vi "Autonomous Independent.vi"() -> ()   [LabVIEW 2016]
doc: "This VI is called when autonomous begins, and will automatically be terminated when autonomous ends. You can carry out timed or sensor driven robot movement independently without needing to return to the caller."
uses:
  <vilib>/Rock Robotics/WPI/Solenoid/WPI_SolenoidValue.ctl
  <vilib>/Rock Robotics/WPI/Utilities/WPI_GetSetVariantRefNum.vi
  <vilib>/Rock Robotics/Network Tables/NT Write Numeric Array.vi
  <vilib>/Rock Robotics/Network Tables/NT Read String.vi
  <vilib>/Rock Robotics/WPI/Solenoid/WPI_SolenoidSetEnum.vi
  <vilib>/addons/control/pid/pid.llb/PID (DBL).vi
  <vilib>/Rock Robotics/WPI/RobotDrive/WPI_RobotDriveMecanumDrive_Cartesian.vi
  <vilib>/Rock Robotics/Network Tables/NT Read Number.vi
  <vilib>/addons/control/pid/NI_PID_pid.lvlib
panel:
  out "Elapsed Time (s) 3":dbl caption="Elapsed Time (s)"
  out "Time has Elapsed 3":bool caption="Time has Elapsed"
  out "s? t:f 3":dbl=0.9
  out "x .or. y? 3":bool=TRUE
  in  "speed 3":dbl(slide)=0.10126903553299492 scale=-0.15..0.15
  in  "setpoint 3":dbl(slide) scale=-50.0..50.0
  in  "PID gains 3":T1={"proportional gain (Kc)"=1.0, "integral time (Ti, min)"=0.01, "derivative time (Td, min)"=0.0} {"derivative time (Td, min)" scale=0.0..0.05; "integral time (Ti, min)" scale=0.0..0.00243; "proportional gain (Kc)" scale=0.0..0.284195}
  out "proportional gain (Kc) 3":dbl=1.0
  out "integral time (Ti, min) 3":dbl=0.01
  out "derivative time (Td, min) 3":dbl
  out "substitute 3":bool
  out "STOP? 3":bool
  out "limit of sensor dist 3":dbl
  out "Current Movement, for debugging":T2 {"Z Joystick Value" scale=-1.0..1.0; "Y Joystick Value" scale=1.0..-1.0; "X Joystick Value" scale=-1.0..1.0}
  in  "Array of robot movements":T3(array[cluster])=[{"X Joystick Value"=-0.010101010101010017, "Y Joystick Value"=0.0, "Z Joystick Value"=0.4574773480918073, "Delay (sec)"=0.0, "Movement Name"=""}, {"X Joystick Value"=0.050505050505050594, "Y Joystick Value"=0.0, "Z Joystick Value"=-0.25616029503917137, "Delay (sec)"=0.0, "Movement Name"=""}] {"Z Joystick Value" scale=-1.0..1.0; "Y Joystick Value" scale=1.0..-1.0; "X Joystick Value" scale=-1.0..1.0}
  out "Elapsed Time (s) 2":dbl caption="Elapsed Time (s)"
  out "Time has Elapsed 2":bool caption="Time has Elapsed"
  out "s? t:f 2":dbl=0.9
  out "x .or. y? 2":bool=TRUE
  in  "speed 2":dbl(slide)=0.10126903553299492 scale=-0.15..0.15
  in  "setpoint 2":dbl(slide) scale=-50.0..50.0
  in  "PID gains 2":T1={"proportional gain (Kc)"=1.0, "integral time (Ti, min)"=0.01, "derivative time (Td, min)"=0.0} {"derivative time (Td, min)" scale=0.0..0.05; "integral time (Ti, min)" scale=0.0..0.00243; "proportional gain (Kc)" scale=0.0..0.284195}
  out "proportional gain (Kc) 2":dbl=1.0
  out "integral time (Ti, min) 2":dbl=0.01
  out "derivative time (Td, min) 2":dbl
  out "substitute 2":bool
  out "STOP? 2":bool
  out "limit of sensor dist 2":dbl
  out "Elapsed Time (s)":dbl
  out "Time has Elapsed":bool
  out "Left":dbl(graph)=57.45456942754214
  out "Right":dbl(graph)=69.75220843172497
  out "s? t:f":dbl=0.9
  out "x .or. y?":bool=TRUE
  in  "speed":dbl(slide)=0.10126903553299492 scale=-0.15..0.15
  out "Yaw":dbl(graph)
  out "Data":T4(graph)={"setpoint"=0.0, "Yaw"=2.26, "dt out (s)"=0.0010000000474974513}
  in  "setpoint":dbl(slide) scale=-50.0..50.0
  in  "PID gains":T1={"proportional gain (Kc)"=1.0, "integral time (Ti, min)"=0.01, "derivative time (Td, min)"=0.0} {"derivative time (Td, min)" scale=0.0..0.05; "integral time (Ti, min)" scale=0.0..0.00243; "proportional gain (Kc)" scale=0.0..0.284195}
  out "proportional gain (Kc)":dbl=1.0
  out "integral time (Ti, min)":dbl=0.01
  out "derivative time (Td, min)":dbl
  out "substitute":bool
  out "Right Average":cluster{dbl}(graph)
  out "Left Average":cluster{dbl}(graph)
  out "STOP?":bool
  out "limit of sensor dist":dbl
  out "Yaw 2":dbl
  out "Yaw 3":dbl
  # "Be sure to right-click and choose Data Operations>>Make Current Value default if you want to save the array values with the VI"
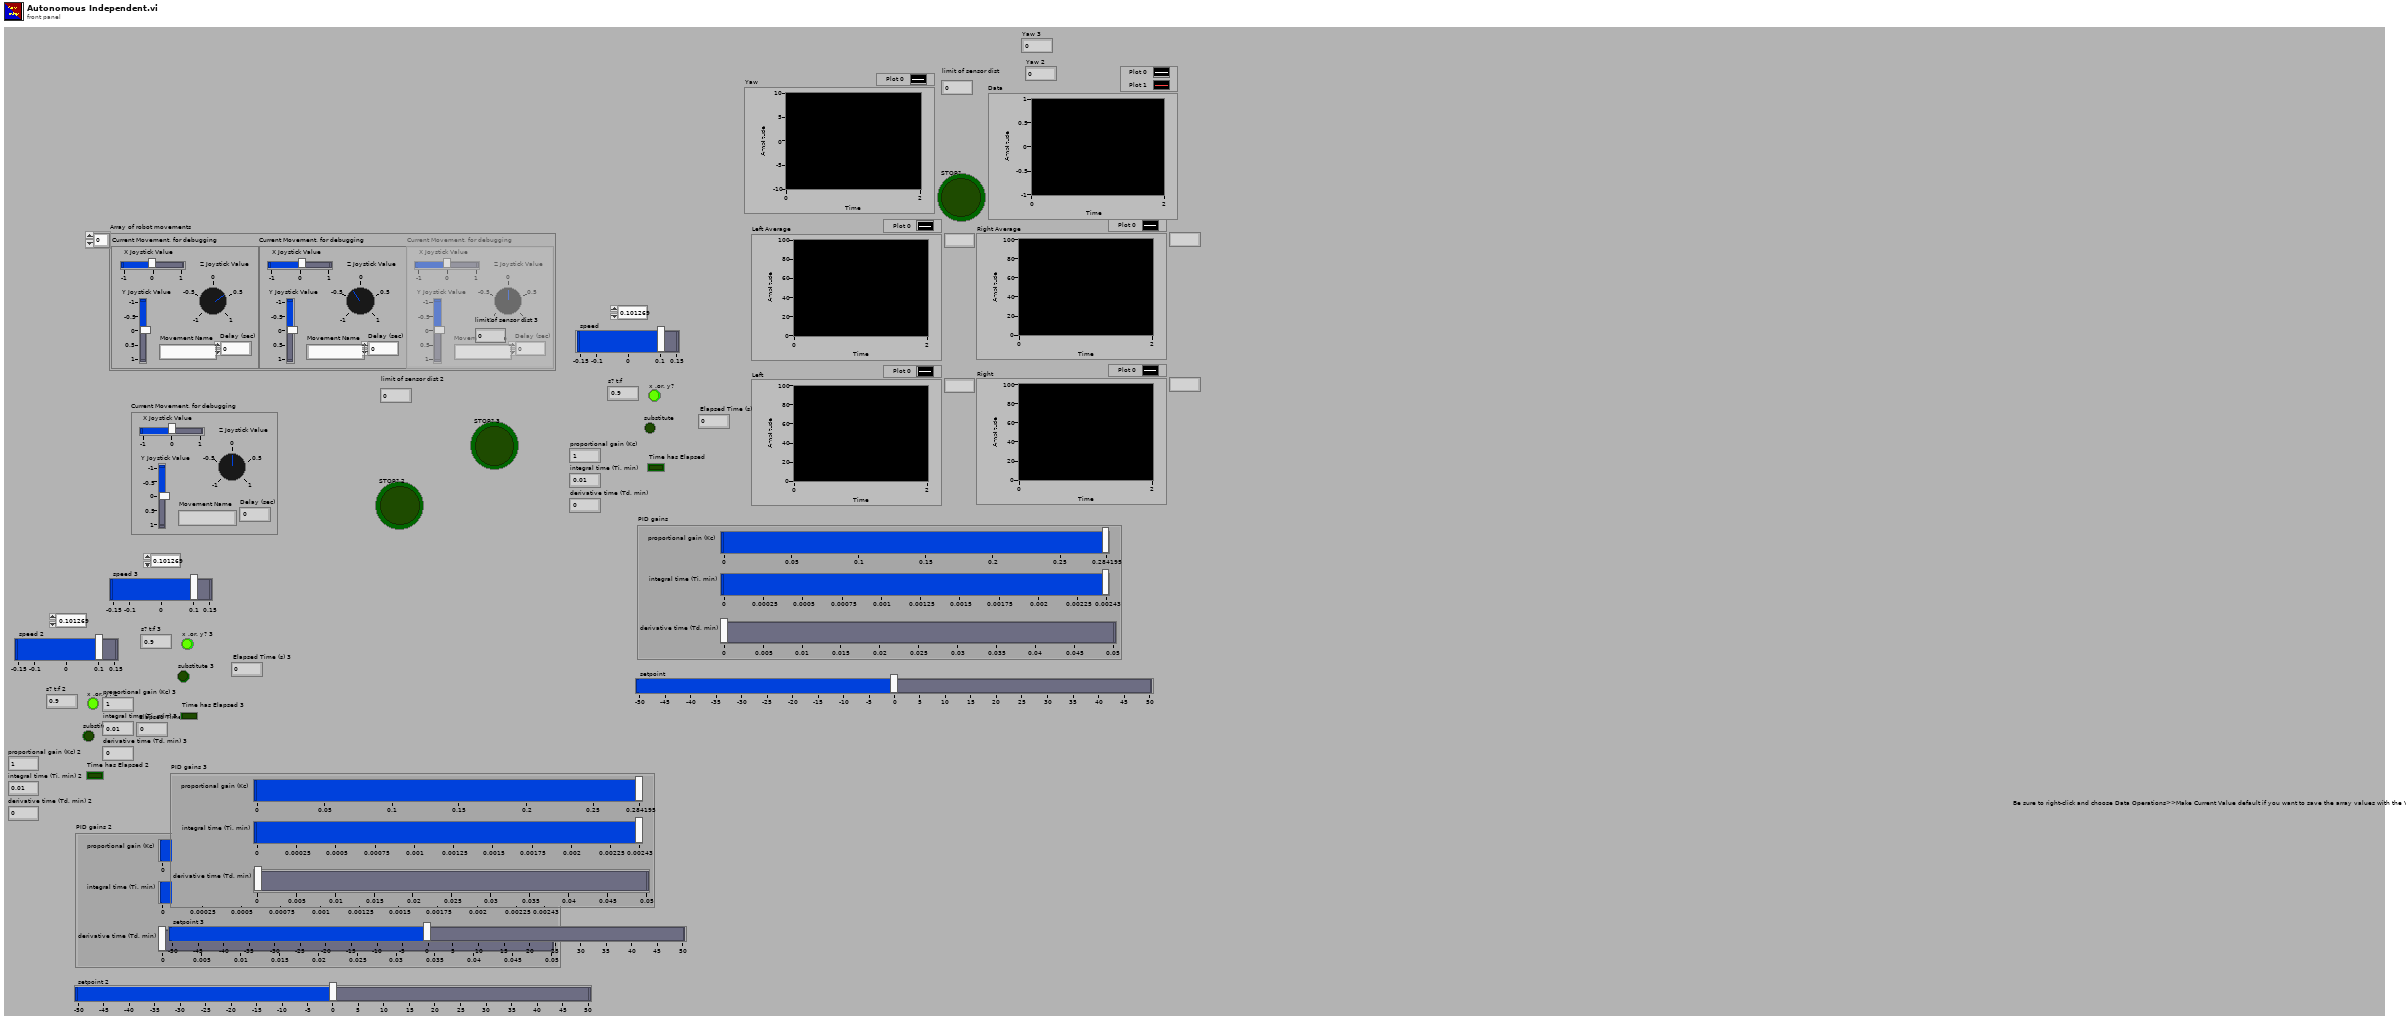
[diagram p1: front panel]
types:
  T1 = cluster{"proportional gain (Kc)":dbl, "integral time (Ti, min)":dbl, "derivative time (Td, min)":dbl}
  T2 = cluster{"X Joystick Value":dbl, "Y Joystick Value":dbl, "Z Joystick Value":dbl, "Delay (sec)":dbl, "Movement Name":string}
  T3 = cluster{"X Joystick Value":dbl, "Y Joystick Value":dbl, "Z Joystick Value":dbl, "Delay (sec)":dbl, "Movement Name":string}[]
  T4 = cluster{"setpoint":dbl, "Yaw":dbl, "dt out (s)":dbl}
  T5 = typedef "WPI_JoystickDevRef.ctl" = cluster{"Device":T6}
  T6 = typedef "WPI_JoystickDeviceEnum.ctl" = enum16{"USB 0", "USB 1", "USB 2", "USB 3", "USB 4", "USB 5"}
  T7 = typedef "WPI_SolenoidValue.ctl" = enum16{"Off", "On", "Forward", "Reverse"}
  T8 = typedef "WPI_SolenoidDevRef.ctl" = cluster{"DevStatus":errorcluster, "Pneumatics Control Module":u8, "Forward Solenoid Channel":T9, "Reverse Solenoid Channel":T9}
  T9 = typedef "WPI_SolenoidChannel.ctl" = enum8{"Solenoid 0", "Solenoid 1", "Solenoid 2", "Solenoid 3", "Solenoid 4", "Solenoid 5", "Solenoid 6", "Solenoid 7", "Invalid"}
  T10 = typedef "WPI_AnalogChannelDevRef.ctl" = cluster{"DevStatus":errorcluster, "Analog Channel":T11}
  T11 = typedef "FPGA_AIChannel.ctl" = enum8{"AI 0", "AI 1", "AI 2", "AI 3", "AI MXP 0", "AI MXP 1", "AI MXP 2", "AI MXP 3", "Invalid"}
  T12 = typedef "WPI_RobotDriveDevRef.ctl" = cluster{"DevStatus":errorcluster, "Motors[]":T13[], "Square Inputs":bool, "Max Output":dbl}
  T13 = typedef "WPI_MotorControlDeviceRef.ctl" = cluster{"DeviceStatus":errorcluster, "Type":T14, "PWM":cluster{"PWM Channel":T15, "DeadBand":T16}, "CAN":cluster{"Device Number":u8, "SetOutput VI Ref":variant, "GetOutput VI Ref":variant, "Enable VI Ref":variant, "Disable VI Ref":variant, "Data":variant}, "Invert":bool}
  T14 = typedef "WPI_MotorControlType.ctl" = enum16{"PWM", "CAN"}
  T15 = typedef "FPGA_DIOPWMChannel.ctl" = enum8{"PWM 0", "PWM 1", "PWM 2", "PWM 3", "PWM 4", "PWM 5", "PWM 6", "PWM 7", "PWM 8", "PWM 9", "PWM MXP 0", "PWM MXP 1", "PWM MXP 2", "PWM MXP 3", "PWM MXP 4", "PWM MXP 5", "PWM MXP 6", "PWM MXP 7", "PWM MXP 8", "PWM MXP 9", "Invalid"}
  T16 = typedef "WPI_PWMDeadband.ctl" = cluster{"Name":string, "maxPositivePwm":i32, "minPositivePwm":i32, "centerPwm":i32, "maxNegativePwm":i32, "minNegativePwm":i32, "angularRange":u16}
  T17 = cluster{"Yaw":dbl, "Roll":dbl, "Pitch":dbl, "Heading":dbl, "Fused Heading":dbl}
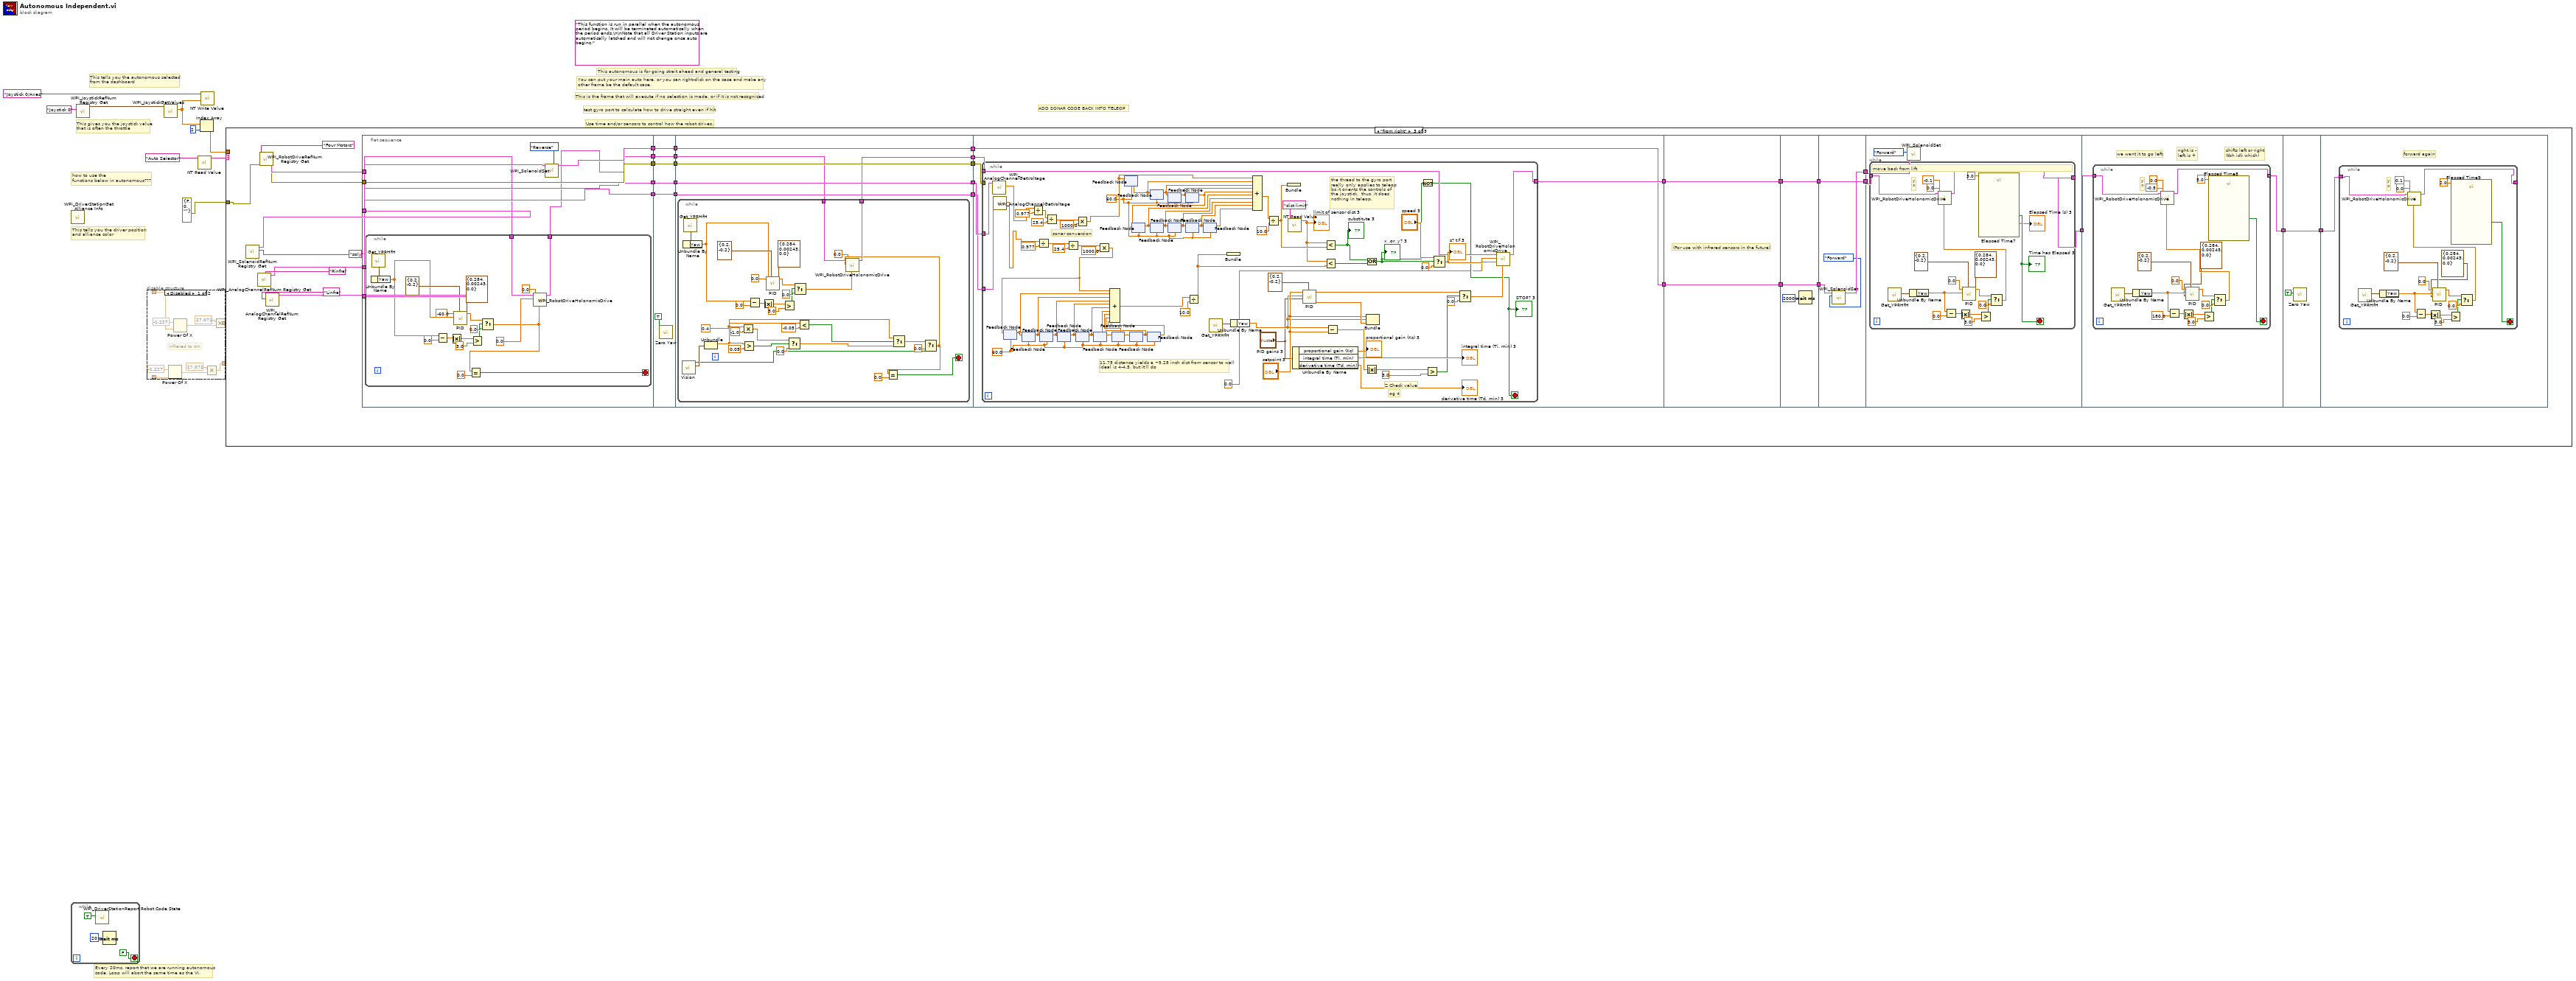
[diagram p0: block diagram]
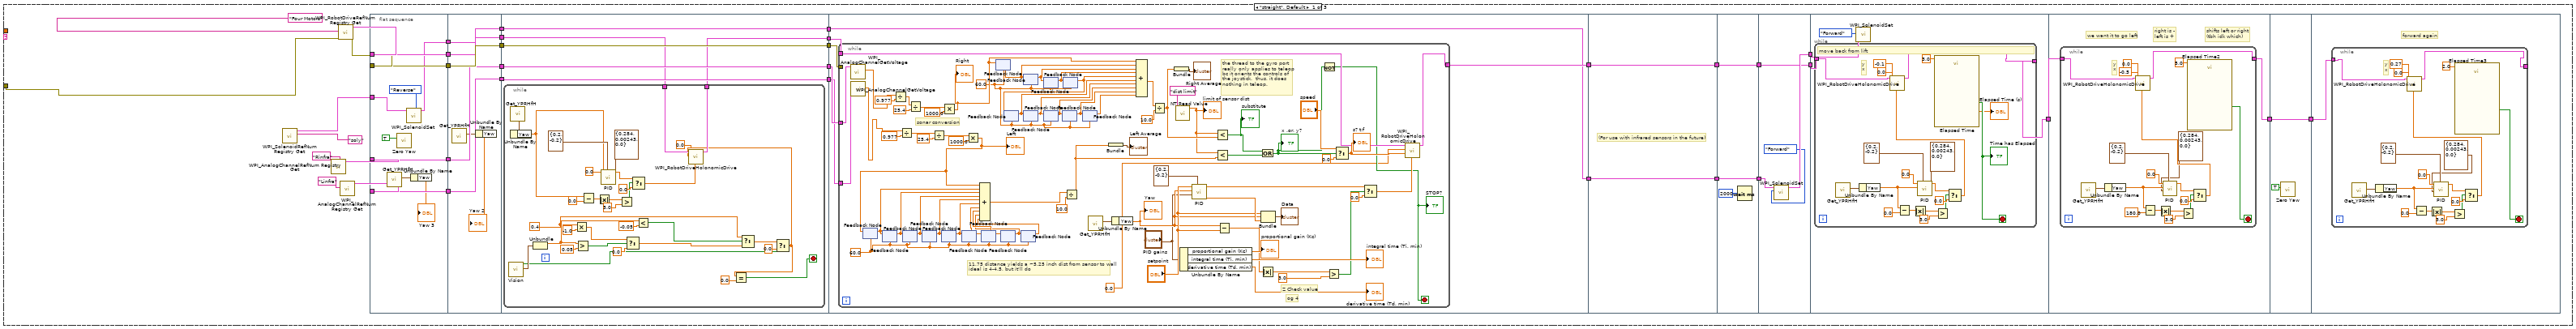
[diagram p3: hidden frame]
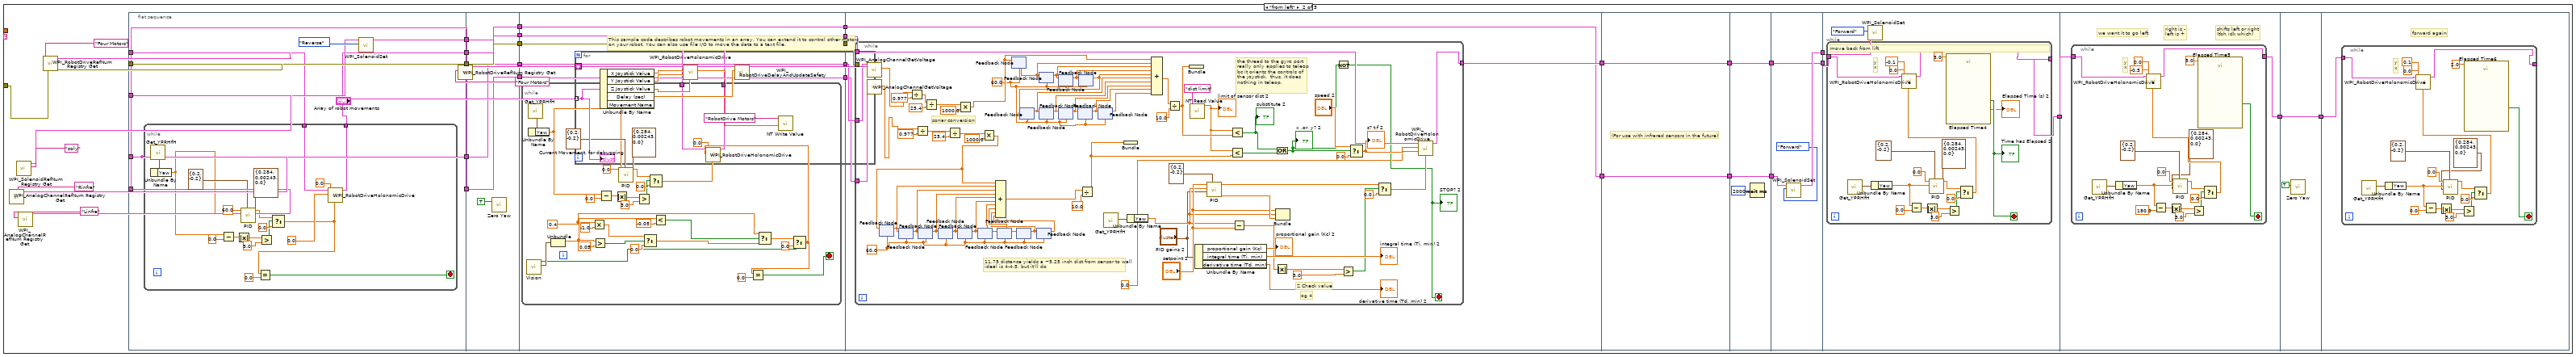
[diagram p4: hidden frame]
diagram:
  (unwired) "This function is run in parallel when the autonomous period begins. It will be terminated automatically when the period ends.\n\nNote that all Driver Station inputs are automatically latched and will not change once auto begins."
  # "ADD SONAR CODE BACK INTO TELEOP"
  # "test gyro port to calculate how to drive straight even if hit"
  # "This autonomous is for going strait ahead and general testing"
  # "You can put your main auto here, or you can right-click on the case and make any\nother frame be the default case."
  # "This is the frame that will execute if no selection is made, or if it is not recognized"
  # "how to use the\nfunctions below in autonomous???"
  # "This tells you the autonomous selected\nfrom the dashboard"
  # "Every 20ms, report that we are running autonomous\ncode. Loop will abort the same time as the VI."
  # "This gives you the joystick value\nthat is often the throttle"
  # "Use time and/or sensors to control how the robot drives."
  # "This tells you the driver position\nand alliance color"
  n1 = call <vilib>:"WPI_DriverStationGet Alliance Info.vi"() -> ()  [unwired: 12 out]
  n2 = while {
    stop <- FALSE stop-if-true
    n3 = call <vilib>:"WPI_DriverStationReport Robot Code State.vi"("Autonomous"=TRUE) -> ()  [unwired: 10 in, 1 out]
    n4 = Wait (ms)(milliseconds to wait=u32 20) -> ()  [unwired: 1 out]
  }
  n5 = call <vilib>:"WPI_JoystickRefNum Registry Get.vi"("refnum name"="Joystick 0") -> ("JoystickDevRef"=w8:T5)  [unwired: 1 in, 9 out]
  n6 = disable-structure shown="Disabled" {
    disable-tunnel: _ -> [w16 _]
    disable-tunnel: _ -> [w15 _]
    disable-tunnel: [w14 _] -> _
    disable-tunnel: [w13 _] -> _
    frame Disabled {
      # "infrared to cm"
      n7 = Power Of X(1:w15, 2:-1.227 ("y")) -> (0:w19:dbl)
      n8 = Power Of X(1:w16, 2:-1.227 ("y")) -> (0:w20:dbl)
      n9 = Multiply(x=27.071, y=w19) -> (x*y=w13:dbl)
      n10 = Multiply(x=27.071, y=w20) -> (x*y=w14:dbl)
    }
    frame Enabled {
    }
  }
  n11 = call <vilib>:"WPI_JoystickGetValues.vi"("JoystickDevRef"=w8) -> ("Axes"=w2:dbl[])  [unwired: 6 in, 4 out]
  n12 = call-poly <vilib>:"NT Read Value.vi"("Name"="Auto Selector") -> ("String"=w5:string)  [unwired: 9 in, 1 out]
  n13 = Index Array(array=w2, index=u32 2 ("milliseconds to wait")) -> (element=w4:dbl)
  n14 = call-poly <vilib>:"NT Write Value.vi"("Numeric Array"=w2, "Name"="Joystick 0/Axes") -> ()  [unwired: 9 in, 1 out]
  n15 = case shown="\"from right\"" w5 {
    tunnel: w4 -> [_ _ _]
    tunnel: errorcluster {"status"=FALSE, "code"=0, "source"=""} ("error in (no error)") -> [w51 w271 w556]
    frame "straight", Default {
      n16 = call <vilib>:"WPI_SolenoidRefNum Registry Get.vi"("refnum name"="soly") -> ("SolenoidDevRef"=w46:T8)  [unwired: 9 in, 1 out]
      n17 = call <vilib>:"WPI_AnalogChannelRefNum Registry Get.vi"("refnum name"="Rinfra") -> ("AIDeviceRef"=w53:T10)  [unwired: 9 in, 1 out]
      n18 = call <vilib>:"WPI_RobotDriveRefNum Registry Get.vi"("error in (no error)"=w51, "refnum name"="Four Motors") -> ("error out"=w52:errorcluster, "RobotDriveDevRef"=w57:T12)  [unwired: 8 out]
      n19 = call <vilib>:"WPI_AnalogChannelRefNum Registry Get.vi"("refnum name"="Linfra") -> ("AIDeviceRef"=w54:T10)  [unwired: 9 in, 1 out]
      n20 = flat-sequence {
        tunnel: w52 -> [w65]
        tunnel: w53 -> [w66]
        tunnel: w54 -> [w67]
        tunnel: w57 -> [w68]
        tunnel: [w68] -> w38
        tunnel: [w67] -> w39
        tunnel: [w66] -> w40
        tunnel: [w65] -> w41
        tunnel: w46 -> [w61]
        tunnel: [w62] -> w37
        tunnel: w41 -> [w75]
        tunnel: [w75] -> w32
        tunnel: w40 -> [w71]
        tunnel: [w71] -> w30
        tunnel: w39 -> [w72]
        tunnel: [w72] -> w28
        tunnel: w38 -> [w74]
        tunnel: [w74] -> w26
        tunnel: w37 -> [w73]
        tunnel: [w73] -> w24
        tunnel: w32 -> [w81]
        tunnel: [w81] -> w31
        tunnel: w30 -> [w80]
        tunnel: [w80] -> w29
        tunnel: w28 -> [w79]
        tunnel: [w79] -> w27
        tunnel: w26 -> [w77]
        tunnel: [w76] -> w25
        tunnel: w24 -> [w78]
        tunnel: [w78] -> w23
        tunnel: [w120] -> w43
        tunnel: w31 -> [w118]
        tunnel: w29 -> [w119]
        tunnel: w27 -> [w117]
        tunnel: w25 -> [w116]
        tunnel: w23 -> [w115]
        tunnel: [w115] -> w42
        tunnel: w43 -> [w195]
        tunnel: [w195] -> w36
        tunnel: w42 -> [w194]
        tunnel: [w194] -> w34
        tunnel: w36 -> [w198]
        tunnel: [w198] -> w35
        tunnel: w34 -> [w197]
        tunnel: [w197] -> w33
        tunnel: [w201] -> w50
        tunnel: [w200] -> w49
        tunnel: w35 -> [w200]
        tunnel: w33 -> [w202]
        tunnel: w50 -> [w203]
        tunnel: w49 -> [w206]
        tunnel: [w205] -> w48
        tunnel: w48 -> [w228]
        tunnel: [w227] -> w45
        tunnel: w45 -> [w249]
        tunnel: [w249] -> w44
        tunnel: w44 -> [w250]
        frame #0 {
          n21 = call <vilib>:"Get_YPRHfH.vi"() -> ("YRPHfH"=w60:T17)  [unwired: 11 in]
          n22 = call <vilib>:"Zero Yaw.vi"("Zero"=TRUE) -> ()  [unwired: 11 in]
          n23 = call-poly <vilib>:"WPI_SolenoidSet.vi"("Value"=WPI_SolenoidValue."Reverse", "SolenoidDevRef"=w61) -> ("SolenoidDevRef"=w62:T8)  [unwired: 8 in, 1 out]
          n24 = Unbundle By Name(w60) -> ("Yaw"=→"Yaw 3":dbl)
        }
        frame #1 {
          n25 = call <vilib>:"Get_YPRHfH.vi"() -> ("YRPHfH"=w70:T17)  [unwired: 11 in]
          n26 = Unbundle By Name(w70) -> ("Yaw"=→"Yaw 2":dbl)
        }
        frame #2 {
          n27 = while {
            tunnel: w77 -> [w98]
            tunnel: [w97] -> w76
            stop <- w99 stop-if-true
            w107 = 0.4 ("t")
            n28 = call "Vision.vi"() -> ("Center"=w104:cluster{dbl, dbl}, "seen"=w101:bool)  [unwired: 10 in]
            n29 = call <vilib>:"Get_YPRHfH.vi"() -> ("YRPHfH"=w92:T17)  [unwired: 11 in]
            n30 = Unbundle By Name(w92) -> ("Yaw"=w91:dbl)
            n31 = Unbundle(w104) -> (w114:dbl)  [unwired: 1 out]
            n32 = Multiply(x=w107, y=-1.0) -> (x*y=w108:dbl)
            n33 = Greater?(x=w114, y=0.05) -> (0:w106:bool)
            n34 = Subtract(x=w91, y=0.0) -> (x-y=w89:dbl)
            n35 = Absolute Value(x=w89) -> (abs(x)=w88:dbl)
            n36 = call-poly <vilib>:"PID.vi"("output range"=cluster{"output high":dbl, "output low":dbl} {"output high"=0.2, "output low"=-0.2}, "PID gains"=T1 {"proportional gain (Kc)"=0.284, "integral time (Ti, min)"=0.00243, "derivative time (Td, min)"=0.0}, "process variable"=w91, "setpoint"=0.0) -> ("output"=w85:dbl)  [unwired: 6 in, 1 out]
            n37 = Greater?(x=w88, y=3.0) -> (0:w86:bool)
            n38 = Select(t=w108, s=w106, f=0.0) -> (s? t:f=w112:dbl)
            n39 = Select(t=w85, s=w86, f=0.0) -> (s? t:f=w83:dbl)
            n40 = Less?(x=w114, y=-0.05) -> (x < y?=w105:bool)
            n41 = Select(t=w107, s=w105, f=w112) -> (s? t:f=w103:dbl)
            n42 = Select(t=w103, s=w101, f=0.0) -> (s? t:f=w96:dbl)
            n43 = call-poly <vilib>:"WPI_RobotDriveHolonomicDrive.vi"("Rotation"=w83, "Y"=0.0, "X"=w96, "RobotDriveDevRef"=w98) -> ("RobotDriveDevRef"=w97:T12)  [unwired: 5 in, 2 out]
            n44 = Equal?(x=w96, y=0.0) -> (x = y?=w99:bool)
          }
        }
        frame #3 {
          n45 = while {
            tunnel: w117 -> [w193]
            tunnel: w119 -> [w192]
            tunnel: w118 -> [_]
            tunnel: [w169] -> w120
            tunnel: w116 -> [w168]
            stop <- w126 stop-if-true
            w124 = 60.0
            w125 = 60.0
            # "11.75 distance yields a ~5.25 inch dist from sensor to wall\nideal is 4-4.5, but it'll do"
            # "sonar conversion"
            # "og 4"
            # "the thread to the gyro port\nreally only applies to teleop \nbc it orients the controls of \nthe joystick.  thus, it does \nnothing in teleop."
            # "Z Check value"
            n46 = call <vilib>:"WPI_AnalogChannelGetVoltage.vi"("AIDeviceRef"=w192) -> ("Voltage"=w128:dbl)  [unwired: 8 in, 2 out]
            n47 = call <vilib>:"WPI_AnalogChannelGetVoltage.vi"("AIDeviceRef"=w193) -> ("Voltage"=w129:dbl)  [unwired: 8 in, 2 out]
            n48 = feedback #1(w125) -> (w159:dbl)
            n49 = feedback #2(w125) -> (w158:dbl)
            n50 = feedback-in #2(w159) -> ()
            n51 = Divide(x=w128, y=0.977) -> (x/y=w139:dbl)
            n52 = Divide(x=w129, y=0.977) -> (x/y=w132:dbl)
            n53 = feedback #3(w125) -> (w155:dbl)
            n54 = feedback-in #3(w158) -> ()
            n55 = Divide(x=w139, y=25.4) -> (x/y=w137:dbl)
            n56 = feedback #4(w125) -> (w153:dbl)
            n57 = feedback-in #4(w155) -> ()
            n58 = Divide(x=w132, y=25.4) -> (x/y=w134:dbl)
            n59 = feedback #5(w125) -> (w152:dbl)
            n60 = feedback-in #5(w153) -> ()
            n61 = Multiply(x=w137, y=1000.0) -> (x*y=w130:dbl)
            "Right" <- w130
            n62 = feedback #6(w125) -> (w151:dbl)
            n63 = feedback-in #6(w152) -> ()
            n64 = Multiply(x=w134, y=1000.0) -> (x*y=w127:dbl)
            "Left" <- w127
            n65 = feedback-in #1(w127) -> ()
            n66 = feedback #7(w125) -> (w150:dbl)
            n67 = feedback-in #7(w151) -> ()
            n68 = feedback #8(w124) -> (w166:dbl)
            n69 = feedback-in #8(w130) -> ()
            n70 = feedback #9(w125) -> (w149:dbl)
            n71 = feedback-in #9(w150) -> ()
            n72 = feedback #10(w124) -> (w146:dbl)
            n73 = feedback #11(w125) -> (w148:dbl)
            n74 = Compound Arithmetic op=ADD(w127, w159, w158, w155, w153, w152, w151, w150, w149, w148) -> (w157:dbl)
            n75 = feedback-in #11(w149) -> ()
            n76 = feedback #12(w124) -> (w165:dbl)
            n77 = feedback-in #12(w166) -> ()
            n78 = feedback #13(w124) -> (w145:dbl)
            n79 = feedback-in #13(w146) -> ()
            n80 = feedback #14(w124) -> (w162:dbl)
            n81 = feedback-in #14(w165) -> ()
            n82 = feedback #15(w124) -> (w144:dbl)
            n83 = feedback-in #15(w145) -> ()
            n84 = feedback #16(w124) -> (w143:dbl)
            n85 = feedback-in #16(w144) -> ()
            n86 = feedback #17(w124) -> (w147:dbl)
            n87 = feedback-in #10(w147) -> ()
            n88 = feedback-in #17(w162) -> ()
            n89 = Divide(x=w157, y=10.0) -> (x/y=w154:dbl)
            n90 = feedback #18(w124) -> (w142:dbl)
            n91 = feedback-in #18(w143) -> ()
            n92 = call <vilib>:"Get_YPRHfH.vi"() -> ("YRPHfH"=w180:T17)  [unwired: 11 in]
            n93 = Bundle(w154) -> (→"Left Average":cluster{dbl})  [unwired: 1 in]
            n94 = Unbundle By Name(w180) -> ("Yaw"=w171:dbl)
            "Yaw" <- w171
            n95 = Compound Arithmetic op=ADD(w130, w166, w165, w162, w147, w146, w145, w144, w143, w142) -> (w164:dbl)
            n96 = Divide(x=w164, y=10.0) -> (x/y=w161:dbl)
            n97 = Bundle(w161) -> (→"Right Average":cluster{dbl})  [unwired: 1 in]
            n98 = call-poly <vilib>:"NT Read Value.vi"("Name"="dist limit") -> ("Numeric"=w122:dbl)  [unwired: 9 in, 1 out]
            "limit of sensor dist" <- w122
            n99 = Unbundle By Name("PID gains") -> ("proportional gain (Kc)"=→"proportional gain (Kc)":dbl, "integral time (Ti, min)"=→"integral time (Ti, min)":dbl, "derivative time (Td, min)"=→"derivative time (Td, min)":dbl)
            n100 = call-poly <vilib>:"PID.vi"("output range"=cluster{"output high":dbl, "output low":dbl} {"output high"=0.2, "output low"=-0.2}, "PID gains"="PID gains", "process variable"=w171, "setpoint"="setpoint") -> ("dt out (s)"=w181:dbl, "output"=w182:dbl)  [unwired: 6 in]
            n101 = Less?(x=w122, y=w161) -> (x < y?=w167:bool)
            "substitute" <- w167
            n102 = Less?(x=w122, y=w154) -> (x < y?=w188:bool)
            n103 = Subtract(x=w171, y="setpoint") -> (x-y=w175:dbl)
            n104 = Or(x=w167, y=w188) -> (x .or. y?=w187:bool)
            "x .or. y?" <- w187
            n105 = Absolute Value(x=w175) -> (abs(x)=w173:dbl)
            n106 = Bundle("setpoint"="setpoint", "Yaw"=w171, "dt out (s)"=w181) -> (→"Data":T4)  [unwired: 1 in]
            n107 = Not(x=w187) -> (.not. x?=w126:bool)
            "STOP?" <- w126
            n108 = Greater?(x=w173, y=3.0) -> (0:w176:bool)
            n109 = Select(t="speed", s=w187, f=0.0) -> (s? t:f=w189:dbl)
            "s? t:f" <- w189
            n110 = Select(t=w182, s=w176, f=0.0) -> (s? t:f=w172:dbl)
            n111 = call-poly <vilib>:"WPI_RobotDriveHolonomicDrive.vi"("Rotation"=w172, "Y"=w189, "X"=0.0, "RobotDriveDevRef"=w168) -> ("RobotDriveDevRef"=w169:T12)  [unwired: 5 in, 2 out]
          }
        }
        frame #4 {
          # "(For use with infrared sensors in the future)"
        }
        frame #5 {
          n112 = Wait (ms)(milliseconds to wait=u32 2000) -> ()  [unwired: 1 out]
        }
        frame #6 {
          n113 = call-poly <vilib>:"WPI_SolenoidSet.vi"("Value"=WPI_SolenoidValue."Forward", "SolenoidDevRef"=w202) -> ("SolenoidDevRef"=w201:T8)  [unwired: 8 in, 1 out]
        }
        frame #7 {
          n114 = while {
            tunnel: w206 -> [w212]
            tunnel: [w211] -> w205
            stop <- w208 stop-if-true
            # "y\nx"
            # "move back from lift"
            n115 = call <vilib>:"Get_YPRHfH.vi"() -> ("YRPHfH"=w222:T17)  [unwired: 11 in]
            n116 = Unbundle By Name(w222) -> ("Yaw"=w221:dbl)
            n117 = Subtract(x=w221, y=0.0) -> (x-y=w219:dbl)
            n118 = Absolute Value(x=w219) -> (abs(x)=w218:dbl)
            n119 = call-poly <vilib>:"PID.vi"("output range"=cluster{"output high":dbl, "output low":dbl} {"output high"=0.2, "output low"=-0.2}, "PID gains"=T1 {"proportional gain (Kc)"=0.284, "integral time (Ti, min)"=0.00243, "derivative time (Td, min)"=0.0}, "process variable"=w221, "setpoint"=0.0) -> ("output"=w214:dbl)  [unwired: 6 in, 1 out]
            n120 = call "Elapsed Time"("Time Target (s)"=3.0) -> ("Elapsed Time (s)"=→"Elapsed Time (s)":dbl, "Time has Elapsed"=w208:bool)  [unwired: 11 in, 6 out]
            "Time has Elapsed" <- w208
            n121 = Greater?(x=w218, y=3.0) -> (0:w215:bool)
            n122 = Select(t=w214, s=w215, f=0.0) -> (s? t:f=w213:dbl)
            n123 = call-poly <vilib>:"WPI_RobotDriveHolonomicDrive.vi"("Rotation"=w213, "Y"=-0.1, "X"=0.0, "RobotDriveDevRef"=w212) -> ("RobotDriveDevRef"=w211:T12)  [unwired: 5 in, 2 out]
          }
          n124 = call-poly <vilib>:"WPI_SolenoidSet.vi"("Value"=WPI_SolenoidValue."Forward", "SolenoidDevRef"=w203) -> ()  [unwired: 8 in, 2 out]
        }
        frame #8 {
          # "right is -\nleft is +"
          # "we want it to go left"
          # "shifts left or right\n(tbh idk which)"
          n125 = while {
            tunnel: w228 -> [w233]
            tunnel: [w232] -> w227
            stop <- w229 stop-if-true
            # "y\nx"
            n126 = call <vilib>:"Get_YPRHfH.vi"() -> ("YRPHfH"=w243:T17)  [unwired: 11 in]
            n127 = Unbundle By Name(w243) -> ("Yaw"=w242:dbl)
            n128 = Subtract(x=w242, y=180.0) -> (x-y=w240:dbl)
            n129 = Absolute Value(x=w240) -> (abs(x)=w239:dbl)
            n130 = call-poly <vilib>:"PID.vi"("output range"=cluster{"output high":dbl, "output low":dbl} {"output high"=0.2, "output low"=-0.2}, "PID gains"=T1 {"proportional gain (Kc)"=0.284, "integral time (Ti, min)"=0.00243, "derivative time (Td, min)"=0.0}, "process variable"=w242, "setpoint"=0.0) -> ("output"=w235:dbl)  [unwired: 6 in, 1 out]
            n131 = Greater?(x=w239, y=3.0) -> (0:w236:bool)
            n132 = call "Elapsed Time2"("Time Target (s)"=5.0) -> ("Time has Elapsed"=w229:bool)  [unwired: 11 in, 7 out]
            n133 = Select(t=w235, s=w236, f=0.0) -> (s? t:f=w234:dbl)
            n134 = call-poly <vilib>:"WPI_RobotDriveHolonomicDrive.vi"("Rotation"=w234, "Y"=0.0, "X"=-0.5, "RobotDriveDevRef"=w233) -> ("RobotDriveDevRef"=w232:T12)  [unwired: 5 in, 2 out]
          }
        }
        frame #9 {
          n135 = call <vilib>:"Zero Yaw.vi"("Zero"=TRUE) -> ()  [unwired: 11 in]
        }
        frame #10 {
          # "forward again"
          n136 = while {
            tunnel: w250 -> [w255]
            tunnel: [w254] -> _
            stop <- w251 stop-if-true
            # "y\nx"
            n137 = call <vilib>:"Get_YPRHfH.vi"() -> ("YRPHfH"=w265:T17)  [unwired: 11 in]
            n138 = Unbundle By Name(w265) -> ("Yaw"=w264:dbl)
            n139 = Subtract(x=w264, y=0.0) -> (x-y=w262:dbl)
            n140 = Absolute Value(x=w262) -> (abs(x)=w261:dbl)
            n141 = call-poly <vilib>:"PID.vi"("output range"=cluster{"output high":dbl, "output low":dbl} {"output high"=0.2, "output low"=-0.2}, "PID gains"=T1 {"proportional gain (Kc)"=0.284, "integral time (Ti, min)"=0.00243, "derivative time (Td, min)"=0.0}, "process variable"=w264, "setpoint"=0.0) -> ("output"=w257:dbl)  [unwired: 6 in, 1 out]
            n142 = Greater?(x=w261, y=3.0) -> (0:w258:bool)
            n143 = call "Elapsed Time3"("Time Target (s)"=2.0) -> ("Time has Elapsed"=w251:bool)  [unwired: 11 in, 7 out]
            n144 = Select(t=w257, s=w258, f=0.0) -> (s? t:f=w256:dbl)
            n145 = call-poly <vilib>:"WPI_RobotDriveHolonomicDrive.vi"("Rotation"=w256, "Y"=0.27, "X"=0.0, "RobotDriveDevRef"=w255) -> ("RobotDriveDevRef"=w254:T12)  [unwired: 5 in, 2 out]
          }
        }
      }
    }
    frame "from left" {
      # "This sample code describes robot movements in an array. You can extend it to control other motors\non your robot. You can also use file I/O to move the data to a text file."
      n146 = call <vilib>:"WPI_AnalogChannelRefNum Registry Get.vi"("refnum name"="Rinfra") -> ("AIDeviceRef"=w274:T10)  [unwired: 9 in, 1 out]
      n147 = call <vilib>:"WPI_SolenoidRefNum Registry Get.vi"("refnum name"="soly") -> ("SolenoidDevRef"=w275:T8)  [unwired: 9 in, 1 out]
      n148 = call <vilib>:"WPI_AnalogChannelRefNum Registry Get.vi"("refnum name"="Linfra") -> ("AIDeviceRef"=w273:T10)  [unwired: 9 in, 1 out]
      n149 = call <vilib>:"WPI_RobotDriveRefNum Registry Get.vi"("error in (no error)"=w271, "refnum name"="Four Motors") -> ("error out"=w270:errorcluster, "RobotDriveDevRef"=w272:T12)  [unwired: 8 out]
      n150 = flat-sequence {
        tunnel: w270 -> [w315]
        tunnel: [w311] -> _
        tunnel: w273 -> [w316]
        tunnel: w272 -> [w310]
        tunnel: [w309] -> w302
        tunnel: [w316] -> w303
        tunnel: [w311] -> w304
        tunnel: [w315] -> w305
        tunnel: w275 -> [w312]
        tunnel: [w313] -> w301
        tunnel: w274 -> [w311]
        tunnel: w305 -> [w341]
        tunnel: [w341] -> w300
        tunnel: w304 -> [w337]
        tunnel: [w337] -> w299
        tunnel: w303 -> [w338]
        tunnel: [w338] -> w298
        tunnel: w302 -> [w340]
        tunnel: [w340] -> w297
        tunnel: w301 -> [w339]
        tunnel: [w339] -> w296
        tunnel: w300 -> [w347]
        tunnel: [w347] -> w295
        tunnel: w299 -> [w346]
        tunnel: [w346] -> w294
        tunnel: w298 -> [w345]
        tunnel: [w345] -> w293
        tunnel: w297 -> [w343]
        tunnel: [w342] -> w292
        tunnel: w296 -> [w344]
        tunnel: [w344] -> w291
        tunnel: [w386] -> w290
        tunnel: w295 -> [w384]
        tunnel: w294 -> [w385]
        tunnel: w293 -> [w383]
        tunnel: w292 -> [w382]
        tunnel: w291 -> [w381]
        tunnel: [w381] -> w289
        tunnel: w290 -> [w458]
        tunnel: [w458] -> w288
        tunnel: w289 -> [w457]
        tunnel: [w457] -> w287
        tunnel: w288 -> [w461]
        tunnel: [w461] -> w286
        tunnel: w287 -> [w460]
        tunnel: [w460] -> w285
        tunnel: [w464] -> w284
        tunnel: [w463] -> w283
        tunnel: w286 -> [w463]
        tunnel: w285 -> [w465]
        tunnel: w284 -> [w466]
        tunnel: w283 -> [w469]
        tunnel: [w468] -> w282
        tunnel: w282 -> [w491]
        tunnel: [w490] -> w281
        tunnel: w281 -> [w512]
        tunnel: [w512] -> w280
        tunnel: w280 -> [w513]
        frame #0 {
          n151 = while {
            tunnel: w310 -> [w333]
            tunnel: [w332] -> w309
            stop <- w334 stop-if-true
            n152 = call <vilib>:"Get_YPRHfH.vi"() -> ("YRPHfH"=w328:T17)  [unwired: 11 in]
            n153 = Unbundle By Name(w328) -> ("Yaw"=w327:dbl)
            n154 = Subtract(x=w327, y=0.0) -> (x-y=w325:dbl)
            n155 = Absolute Value(x=w325) -> (abs(x)=w324:dbl)
            n156 = call-poly <vilib>:"PID.vi"("output range"=cluster{"output high":dbl, "output low":dbl} {"output high"=0.2, "output low"=-0.2}, "PID gains"=T1 {"proportional gain (Kc)"=0.284, "integral time (Ti, min)"=0.00243, "derivative time (Td, min)"=0.0}, "process variable"=w327, "setpoint"=60.0) -> ("output"=w321:dbl)  [unwired: 6 in, 1 out]
            n157 = Greater?(x=w324, y=3.0) -> (0:w322:bool)
            n158 = Select(t=w321, s=w322, f=0.0) -> (s? t:f=w317:dbl)
            n159 = Equal?(x=w317, y=0.0) -> (x = y?=w334:bool)
            n160 = call-poly <vilib>:"WPI_RobotDriveHolonomicDrive.vi"("Rotation"=w317, "Y"=0.0, "X"=0.0 ("x"), "RobotDriveDevRef"=w333) -> ("RobotDriveDevRef"=w332:T12)  [unwired: 5 in, 2 out]
          }
          n161 = call-poly <vilib>:"WPI_SolenoidSet.vi"("Value"=WPI_SolenoidValue."Reverse", "SolenoidDevRef"=w312) -> ("SolenoidDevRef"=w313:T8)  [unwired: 8 in, 1 out]
        }
        frame #1 {
          n162 = call <vilib>:"Zero Yaw.vi"("Zero"=TRUE) -> ()  [unwired: 11 in]
        }
        frame #2 {
          n163 = while {
            tunnel: w343 -> [w364]
            tunnel: [w363] -> w342
            stop <- w365 stop-if-true
            w373 = 0.4 ("t")
            n164 = call "Vision.vi"() -> ("Center"=w370:cluster{dbl, dbl}, "seen"=w367:bool)  [unwired: 10 in]
            n165 = call <vilib>:"Get_YPRHfH.vi"() -> ("YRPHfH"=w358:T17)  [unwired: 11 in]
            n166 = Unbundle By Name(w358) -> ("Yaw"=w357:dbl)
            n167 = Unbundle(w370) -> (w380:dbl)  [unwired: 1 out]
            n168 = Multiply(x=w373, y=-1.0) -> (x*y=w374:dbl)
            n169 = Greater?(x=w380, y=0.05) -> (0:w372:bool)
            n170 = Subtract(x=w357, y=0.0) -> (x-y=w355:dbl)
            n171 = Absolute Value(x=w355) -> (abs(x)=w354:dbl)
            n172 = call-poly <vilib>:"PID.vi"("output range"=cluster{"output high":dbl, "output low":dbl} {"output high"=0.2, "output low"=-0.2}, "PID gains"=T1 {"proportional gain (Kc)"=0.284, "integral time (Ti, min)"=0.00243, "derivative time (Td, min)"=0.0}, "process variable"=w357, "setpoint"=0.0) -> ("output"=w351:dbl)  [unwired: 6 in, 1 out]
            n173 = Greater?(x=w354, y=3.0) -> (0:w352:bool)
            n174 = Select(t=w374, s=w372, f=0.0) -> (s? t:f=w378:dbl)
            n175 = Select(t=w351, s=w352, f=0.0) -> (s? t:f=w349:dbl)
            n176 = Less?(x=w380, y=-0.05) -> (x < y?=w371:bool)
            n177 = Select(t=w373, s=w371, f=w378) -> (s? t:f=w369:dbl)
            n178 = Select(t=w369, s=w367, f=0.0) -> (s? t:f=w362:dbl)
            n179 = call-poly <vilib>:"WPI_RobotDriveHolonomicDrive.vi"("Rotation"=w349, "Y"=0.0, "X"=w362, "RobotDriveDevRef"=w364) -> ("RobotDriveDevRef"=w363:T12)  [unwired: 5 in, 2 out]
            n180 = Equal?(x=w362, y=0.0) -> (x = y?=w365:bool)
          }
        }
        frame #3 {
          n181 = while {
            tunnel: w383 -> [w456]
            tunnel: w385 -> [w455]
            tunnel: w384 -> [_]
            tunnel: [w433] -> w386
            tunnel: w382 -> [w432]
            stop <- w392 stop-if-true
            w390 = 60.0
            w391 = 60.0
            # "11.75 distance yields a ~5.25 inch dist from sensor to wall\nideal is 4-4.5, but it'll do"
            # "sonar conversion"
            # "og 4"
            # "the thread to the gyro port\nreally only applies to teleop \nbc it orients the controls of \nthe joystick.  thus, it does \nnothing in teleop."
            # "Z Check value"
            n182 = call <vilib>:"WPI_AnalogChannelGetVoltage.vi"("AIDeviceRef"=w455) -> ("Voltage"=w394:dbl)  [unwired: 8 in, 2 out]
            n183 = call <vilib>:"WPI_AnalogChannelGetVoltage.vi"("AIDeviceRef"=w456) -> ("Voltage"=w395:dbl)  [unwired: 8 in, 2 out]
            n184 = feedback #19(w391) -> (w424:dbl)
            n185 = feedback #20(w391) -> (w423:dbl)
            n186 = feedback-in #20(w424) -> ()
            n187 = Divide(x=w394, y=0.977) -> (x/y=w405:dbl)
            n188 = Divide(x=w395, y=0.977) -> (x/y=w398:dbl)
            n189 = feedback #21(w391) -> (w420:dbl)
            n190 = feedback-in #21(w423) -> ()
            n191 = Divide(x=w405, y=25.4) -> (x/y=w403:dbl)
            n192 = feedback #22(w391) -> (w418:dbl)
            n193 = feedback-in #22(w420) -> ()
            n194 = Divide(x=w398, y=25.4) -> (x/y=w400:dbl)
            n195 = feedback #23(w391) -> (w417:dbl)
            n196 = feedback-in #23(w418) -> ()
            n197 = Multiply(x=w403, y=1000.0) -> (x*y=w396:dbl)
            n198 = feedback #24(w391) -> (w416:dbl)
            n199 = feedback-in #24(w417) -> ()
            n200 = Multiply(x=w400, y=1000.0) -> (x*y=w393:dbl)
            n201 = feedback-in #19(w393) -> ()
            n202 = feedback #25(w391) -> (w415:dbl)
            n203 = feedback-in #25(w416) -> ()
            n204 = feedback #26(w390) -> (w430:dbl)
            n205 = feedback-in #26(w396) -> ()
            n206 = feedback #27(w391) -> (w414:dbl)
            n207 = feedback-in #27(w415) -> ()
            n208 = feedback #28(w390) -> (w411:dbl)
            n209 = feedback #29(w391) -> (w413:dbl)
            n210 = Compound Arithmetic op=ADD(w393, w424, w423, w420, w418, w417, w416, w415, w414, w413) -> (w422:dbl)
            n211 = feedback-in #29(w414) -> ()
            n212 = feedback #30(w390) -> (w429:dbl)
            n213 = feedback-in #30(w430) -> ()
            n214 = feedback #31(w390) -> (w410:dbl)
            n215 = feedback-in #31(w411) -> ()
            n216 = feedback #32(w390) -> (w426:dbl)
            n217 = feedback-in #32(w429) -> ()
            n218 = feedback #33(w390) -> (w409:dbl)
            n219 = feedback-in #33(w410) -> ()
            n220 = feedback #34(w390) -> (w408:dbl)
            n221 = feedback-in #34(w409) -> ()
            n222 = feedback #35(w390) -> (w412:dbl)
            n223 = feedback-in #28(w412) -> ()
            n224 = feedback-in #35(w426) -> ()
            n225 = Divide(x=w422, y=10.0) -> (x/y=w419:dbl)
            n226 = feedback #36(w390) -> (w407:dbl)
            n227 = feedback-in #36(w408) -> ()
            n228 = call <vilib>:"Get_YPRHfH.vi"() -> ("YRPHfH"=w443:T17)  [unwired: 11 in]
            n229 = Bundle(w419) -> ()  [unwired: 1 in, 1 out]
            n230 = Unbundle By Name(w443) -> ("Yaw"=w435:dbl)
            n231 = Compound Arithmetic op=ADD(w396, w430, w429, w426, w412, w411, w410, w409, w408, w407) -> (w428:dbl)
            n232 = Divide(x=w428, y=10.0) -> (x/y=w425:dbl)
            n233 = Bundle(w425) -> ()  [unwired: 1 in, 1 out]
            n234 = call-poly <vilib>:"NT Read Value.vi"("Name"="dist limit") -> ("Numeric"=w388:dbl)  [unwired: 9 in, 1 out]
            "limit of sensor dist 2" <- w388
            n235 = Unbundle By Name("PID gains 2") -> ("proportional gain (Kc)"=→"proportional gain (Kc) 2":dbl, "integral time (Ti, min)"=→"integral time (Ti, min) 2":dbl, "derivative time (Td, min)"=→"derivative time (Td, min) 2":dbl)
            n236 = call-poly <vilib>:"PID.vi"("output range"=cluster{"output high":dbl, "output low":dbl} {"output high"=0.2, "output low"=-0.2}, "PID gains"="PID gains 2", "process variable"=w435, "setpoint"="setpoint 2") -> ("dt out (s)"=w444:dbl, "output"=w445:dbl)  [unwired: 6 in]
            n237 = Less?(x=w388, y=w425) -> (x < y?=w431:bool)
            "substitute 2" <- w431
            n238 = Less?(x=w388, y=w419) -> (x < y?=w451:bool)
            n239 = Subtract(x=w435, y="setpoint 2") -> (x-y=w439:dbl)
            n240 = Or(x=w431, y=w451) -> (x .or. y?=w450:bool)
            "x .or. y? 2" <- w450
            n241 = Absolute Value(x=w439) -> (abs(x)=w437:dbl)
            n242 = Bundle("setpoint 2"="setpoint 2", "Yaw"=w435, "dt out (s)"=w444) -> ()  [unwired: 1 in, 1 out]
            n243 = Not(x=w450) -> (.not. x?=w392:bool)
            "STOP? 2" <- w392
            n244 = Greater?(x=w437, y=3.0) -> (0:w440:bool)
            n245 = Select(t="speed 2", s=w450, f=0.0) -> (s? t:f=w452:dbl)
            "s? t:f 2" <- w452
            n246 = Select(t=w445, s=w440, f=0.0) -> (s? t:f=w436:dbl)
            n247 = call-poly <vilib>:"WPI_RobotDriveHolonomicDrive.vi"("Rotation"=w436, "Y"=w452, "X"=0.0, "RobotDriveDevRef"=w432) -> ("RobotDriveDevRef"=w433:T12)  [unwired: 5 in, 2 out]
          }
        }
        frame #4 {
          # "(For use with infrared sensors in the future)"
        }
        frame #5 {
          n248 = Wait (ms)(milliseconds to wait=u32 2000) -> ()  [unwired: 1 out]
        }
        frame #6 {
          n249 = call-poly <vilib>:"WPI_SolenoidSet.vi"("Value"=WPI_SolenoidValue."Forward", "SolenoidDevRef"=w465) -> ("SolenoidDevRef"=w464:T8)  [unwired: 8 in, 1 out]
        }
        frame #7 {
          n250 = while {
            tunnel: w469 -> [w475]
            tunnel: [w474] -> w468
            stop <- w471 stop-if-true
            # "y\nx"
            # "move back from lift"
            n251 = call <vilib>:"Get_YPRHfH.vi"() -> ("YRPHfH"=w485:T17)  [unwired: 11 in]
            n252 = Unbundle By Name(w485) -> ("Yaw"=w484:dbl)
            n253 = Subtract(x=w484, y=0.0) -> (x-y=w482:dbl)
            n254 = Absolute Value(x=w482) -> (abs(x)=w481:dbl)
            n255 = call-poly <vilib>:"PID.vi"("output range"=cluster{"output high":dbl, "output low":dbl} {"output high"=0.2, "output low"=-0.2}, "PID gains"=T1 {"proportional gain (Kc)"=0.284, "integral time (Ti, min)"=0.00243, "derivative time (Td, min)"=0.0}, "process variable"=w484, "setpoint"=0.0) -> ("output"=w477:dbl)  [unwired: 6 in, 1 out]
            n256 = call "Elapsed Time4"("Time Target (s)"=3.0) -> ("Elapsed Time (s)"=→"Elapsed Time (s) 2":dbl, "Time has Elapsed"=w471:bool)  [unwired: 11 in, 6 out]
            "Time has Elapsed 2" <- w471
            n257 = Greater?(x=w481, y=3.0) -> (0:w478:bool)
            n258 = Select(t=w477, s=w478, f=0.0) -> (s? t:f=w476:dbl)
            n259 = call-poly <vilib>:"WPI_RobotDriveHolonomicDrive.vi"("Rotation"=w476, "Y"=-0.1, "X"=0.0, "RobotDriveDevRef"=w475) -> ("RobotDriveDevRef"=w474:T12)  [unwired: 5 in, 2 out]
          }
          n260 = call-poly <vilib>:"WPI_SolenoidSet.vi"("Value"=WPI_SolenoidValue."Forward", "SolenoidDevRef"=w466) -> ()  [unwired: 8 in, 2 out]
        }
        frame #8 {
          # "right is -\nleft is +"
          # "we want it to go left"
          # "shifts left or right\n(tbh idk which)"
          n261 = while {
            tunnel: w491 -> [w496]
            tunnel: [w495] -> w490
            stop <- w492 stop-if-true
            # "y\nx"
            n262 = call <vilib>:"Get_YPRHfH.vi"() -> ("YRPHfH"=w506:T17)  [unwired: 11 in]
            n263 = Unbundle By Name(w506) -> ("Yaw"=w505:dbl)
            n264 = Subtract(x=w505, y=180.0) -> (x-y=w503:dbl)
            n265 = Absolute Value(x=w503) -> (abs(x)=w502:dbl)
            n266 = call-poly <vilib>:"PID.vi"("output range"=cluster{"output high":dbl, "output low":dbl} {"output high"=0.2, "output low"=-0.2}, "PID gains"=T1 {"proportional gain (Kc)"=0.284, "integral time (Ti, min)"=0.00243, "derivative time (Td, min)"=0.0}, "process variable"=w505, "setpoint"=0.0) -> ("output"=w498:dbl)  [unwired: 6 in, 1 out]
            n267 = Greater?(x=w502, y=3.0) -> (0:w499:bool)
            n268 = call "Elapsed Time5"("Time Target (s)"=5.0) -> ("Time has Elapsed"=w492:bool)  [unwired: 11 in, 7 out]
            n269 = Select(t=w498, s=w499, f=0.0) -> (s? t:f=w497:dbl)
            n270 = call-poly <vilib>:"WPI_RobotDriveHolonomicDrive.vi"("Rotation"=w497, "Y"=0.0, "X"=-0.5, "RobotDriveDevRef"=w496) -> ("RobotDriveDevRef"=w495:T12)  [unwired: 5 in, 2 out]
          }
        }
        frame #9 {
          n271 = call <vilib>:"Zero Yaw.vi"("Zero"=TRUE) -> ()  [unwired: 11 in]
        }
        frame #10 {
          # "forward again"
          n272 = while {
            tunnel: w513 -> [w518]
            tunnel: [w517] -> _
            stop <- w514 stop-if-true
            # "y\nx"
            n273 = call <vilib>:"Get_YPRHfH.vi"() -> ("YRPHfH"=w528:T17)  [unwired: 11 in]
            n274 = Unbundle By Name(w528) -> ("Yaw"=w527:dbl)
            n275 = Subtract(x=w527, y=0.0) -> (x-y=w525:dbl)
            n276 = Absolute Value(x=w525) -> (abs(x)=w524:dbl)
            n277 = call-poly <vilib>:"PID.vi"("output range"=cluster{"output high":dbl, "output low":dbl} {"output high"=0.2, "output low"=-0.2}, "PID gains"=T1 {"proportional gain (Kc)"=0.284, "integral time (Ti, min)"=0.00243, "derivative time (Td, min)"=0.0}, "process variable"=w527, "setpoint"=0.0) -> ("output"=w520:dbl)  [unwired: 6 in, 1 out]
            n278 = Greater?(x=w524, y=3.0) -> (0:w521:bool)
            n279 = call "Elapsed Time6"("Time Target (s)"=2.0) -> ("Time has Elapsed"=w514:bool)  [unwired: 11 in, 7 out]
            n280 = Select(t=w520, s=w521, f=0.0) -> (s? t:f=w519:dbl)
            n281 = call-poly <vilib>:"WPI_RobotDriveHolonomicDrive.vi"("Rotation"=w519, "Y"=0.1, "X"=0.0, "RobotDriveDevRef"=w518) -> ("RobotDriveDevRef"=w517:T12)  [unwired: 5 in, 2 out]
          }
        }
      }
      n282 = call <vilib>:"WPI_RobotDriveRefNum Registry Get.vi"("refnum name"="Four Motors") -> ("RobotDriveDevRef"=w307:T12)  [unwired: 1 in, 9 out]
      n283 = for {
        shift-right: [w540] -> _
        shift-left: w307 -> [w541]
        tunnel: "Array of robot movements" -> [w536] mode=indexing
        n284 = Unbundle By Name(w536) -> ("X Joystick Value"=w539:dbl, "Y Joystick Value"=w538:dbl, "Z Joystick Value"=w535:dbl, "Delay (sec)"=w537:dbl)  [unwired: 1 out]
        n285 = call-poly <vilib>:"WPI_RobotDriveHolonomicDrive.vi"("Rotation"=w535, "Y"=w538, "X"=w539, "RobotDriveDevRef"=w541) -> ("Motor Values"=w533:dbl[], "RobotDriveDevRef"=w542:T12)  [unwired: 5 in, 1 out]
        n286 = call <vilib>:"WPI_RobotDriveDelayAndUpdateSafety.vi"("Delay (s)"=w537, "RobotDriveDevRef"=w542) -> ("RobotDriveDevRef 2"=w540:T12)  [unwired: 8 in, 1 out]
        n287 = call-poly <vilib>:"NT Write Value.vi"("Numeric Array"=w533, "Name"="RobotDrive Motors") -> ()  [unwired: 9 in, 1 out]
        "Current Movement, for debugging" <- w536
      }
    }
    frame "from right" {
      n288 = call <vilib>:"WPI_SolenoidRefNum Registry Get.vi"("refnum name"="soly") -> ("SolenoidDevRef"=w555:T8)  [unwired: 9 in, 1 out]
      n289 = call <vilib>:"WPI_AnalogChannelRefNum Registry Get.vi"("refnum name"="Rinfra") -> ("AIDeviceRef"=w554:T10)  [unwired: 9 in, 1 out]
      n290 = call <vilib>:"WPI_RobotDriveRefNum Registry Get.vi"("error in (no error)"=w556, "refnum name"="Four Motors") -> ("error out"=w557:errorcluster, "RobotDriveDevRef"=w558:T12)  [unwired: 8 out]
      n291 = call <vilib>:"WPI_AnalogChannelRefNum Registry Get.vi"("refnum name"="Linfra") -> ("AIDeviceRef"=w553:T10)  [unwired: 9 in, 1 out]
      n292 = flat-sequence {
        tunnel: [w586] -> w552
        tunnel: [w583] -> w550
        tunnel: [w584] -> w548
        tunnel: [w579] -> w546
        tunnel: [w585] -> w544
        tunnel: w555 -> [w581]
        tunnel: w557 -> [w586]
        tunnel: w554 -> [w583]
        tunnel: w553 -> [w584]
        tunnel: w558 -> [w580]
        tunnel: w552 -> [w611]
        tunnel: [w611] -> w551
        tunnel: w550 -> [w610]
        tunnel: [w610] -> w549
        tunnel: w548 -> [w609]
        tunnel: [w609] -> w547
        tunnel: w546 -> [w608]
        tunnel: [w608] -> w545
        tunnel: w544 -> [w607]
        tunnel: [w607] -> w543
        tunnel: w551 -> [w617]
        tunnel: [w617] -> w578
        tunnel: w549 -> [w616]
        tunnel: [w616] -> w577
        tunnel: w547 -> [w615]
        tunnel: [w615] -> w576
        tunnel: w545 -> [w613]
        tunnel: [w612] -> w575
        tunnel: w543 -> [w614]
        tunnel: [w614] -> w574
        tunnel: [w656] -> w573
        tunnel: w578 -> [w654]
        tunnel: w577 -> [w655]
        tunnel: w576 -> [w653]
        tunnel: w575 -> [w652]
        tunnel: w574 -> [w651]
        tunnel: [w651] -> w572
        tunnel: w573 -> [w728]
        tunnel: [w728] -> w571
        tunnel: w572 -> [w727]
        tunnel: [w727] -> w570
        tunnel: w571 -> [w731]
        tunnel: [w731] -> w569
        tunnel: w570 -> [w730]
        tunnel: [w730] -> w568
        tunnel: [w734] -> w567
        tunnel: [w733] -> w566
        tunnel: w569 -> [w733]
        tunnel: w568 -> [w735]
        tunnel: w567 -> [w736]
        tunnel: w566 -> [w739]
        tunnel: [w738] -> w565
        tunnel: w565 -> [w761]
        tunnel: [w760] -> w564
        tunnel: w564 -> [w782]
        tunnel: [w782] -> w563
        tunnel: w563 -> [w783]
        frame #0 {
          n293 = while {
            tunnel: w580 -> [w603]
            tunnel: [w602] -> w579
            stop <- w604 stop-if-true
            n294 = call <vilib>:"Get_YPRHfH.vi"() -> ("YRPHfH"=w598:T17)  [unwired: 11 in]
            n295 = Unbundle By Name(w598) -> ("Yaw"=w597:dbl)
            n296 = Subtract(x=w597, y=0.0) -> (x-y=w595:dbl)
            n297 = Absolute Value(x=w595) -> (abs(x)=w594:dbl)
            n298 = call-poly <vilib>:"PID.vi"("output range"=cluster{"output high":dbl, "output low":dbl} {"output high"=0.2, "output low"=-0.2}, "PID gains"=T1 {"proportional gain (Kc)"=0.284, "integral time (Ti, min)"=0.00243, "derivative time (Td, min)"=0.0}, "process variable"=w597, "setpoint"=-60.0) -> ("output"=w591:dbl)  [unwired: 6 in, 1 out]
            n299 = Greater?(x=w594, y=3.0) -> (0:w592:bool)
            n300 = Select(t=w591, s=w592, f=0.0) -> (s? t:f=w587:dbl)
            n301 = Equal?(x=w587, y=0.0) -> (x = y?=w604:bool)
            n302 = call-poly <vilib>:"WPI_RobotDriveHolonomicDrive.vi"("Rotation"=w587, "Y"=0.0, "X"=0.0 ("x"), "RobotDriveDevRef"=w603) -> ("RobotDriveDevRef"=w602:T12)  [unwired: 5 in, 2 out]
          }
          n303 = call-poly <vilib>:"WPI_SolenoidSet.vi"("Value"=WPI_SolenoidValue."Reverse", "SolenoidDevRef"=w581) -> ("SolenoidDevRef"=w585:T8)  [unwired: 8 in, 1 out]
        }
        frame #1 {
          n304 = call <vilib>:"Zero Yaw.vi"("Zero"=TRUE) -> ()  [unwired: 11 in]
        }
        frame #2 {
          n305 = while {
            tunnel: w613 -> [w634]
            tunnel: [w633] -> w612
            stop <- w635 stop-if-true
            w643 = 0.4 ("t")
            n306 = call "Vision.vi"() -> ("Center"=w640:cluster{dbl, dbl}, "seen"=w637:bool)  [unwired: 10 in]
            n307 = call <vilib>:"Get_YPRHfH.vi"() -> ("YRPHfH"=w628:T17)  [unwired: 11 in]
            n308 = Unbundle By Name(w628) -> ("Yaw"=w627:dbl)
            n309 = Unbundle(w640) -> (w650:dbl)  [unwired: 1 out]
            n310 = Multiply(x=w643, y=-1.0) -> (x*y=w644:dbl)
            n311 = Greater?(x=w650, y=0.05) -> (0:w642:bool)
            n312 = Subtract(x=w627, y=0.0) -> (x-y=w625:dbl)
            n313 = Absolute Value(x=w625) -> (abs(x)=w624:dbl)
            n314 = call-poly <vilib>:"PID.vi"("output range"=cluster{"output high":dbl, "output low":dbl} {"output high"=0.2, "output low"=-0.2}, "PID gains"=T1 {"proportional gain (Kc)"=0.284, "integral time (Ti, min)"=0.00243, "derivative time (Td, min)"=0.0}, "process variable"=w627, "setpoint"=0.0) -> ("output"=w621:dbl)  [unwired: 6 in, 1 out]
            n315 = Greater?(x=w624, y=3.0) -> (0:w622:bool)
            n316 = Select(t=w644, s=w642, f=0.0) -> (s? t:f=w648:dbl)
            n317 = Select(t=w621, s=w622, f=0.0) -> (s? t:f=w619:dbl)
            n318 = Less?(x=w650, y=-0.05) -> (x < y?=w641:bool)
            n319 = Select(t=w643, s=w641, f=w648) -> (s? t:f=w639:dbl)
            n320 = Select(t=w639, s=w637, f=0.0) -> (s? t:f=w632:dbl)
            n321 = call-poly <vilib>:"WPI_RobotDriveHolonomicDrive.vi"("Rotation"=w619, "Y"=0.0, "X"=w632, "RobotDriveDevRef"=w634) -> ("RobotDriveDevRef"=w633:T12)  [unwired: 5 in, 2 out]
            n322 = Equal?(x=w632, y=0.0) -> (x = y?=w635:bool)
          }
        }
        frame #3 {
          n323 = while {
            tunnel: w653 -> [w726]
            tunnel: w655 -> [w725]
            tunnel: w654 -> [_]
            tunnel: [w703] -> w656
            tunnel: w652 -> [w702]
            stop <- w662 stop-if-true
            w660 = 60.0
            w661 = 60.0
            # "11.75 distance yields a ~5.25 inch dist from sensor to wall\nideal is 4-4.5, but it'll do"
            # "sonar conversion"
            # "og 4"
            # "the thread to the gyro port\nreally only applies to teleop \nbc it orients the controls of \nthe joystick.  thus, it does \nnothing in teleop."
            # "Z Check value"
            n324 = call <vilib>:"WPI_AnalogChannelGetVoltage.vi"("AIDeviceRef"=w725) -> ("Voltage"=w664:dbl)  [unwired: 8 in, 2 out]
            n325 = call <vilib>:"WPI_AnalogChannelGetVoltage.vi"("AIDeviceRef"=w726) -> ("Voltage"=w665:dbl)  [unwired: 8 in, 2 out]
            n326 = feedback #37(w661) -> (w694:dbl)
            n327 = feedback #38(w661) -> (w693:dbl)
            n328 = feedback-in #38(w694) -> ()
            n329 = Divide(x=w664, y=0.977) -> (x/y=w675:dbl)
            n330 = Divide(x=w665, y=0.977) -> (x/y=w668:dbl)
            n331 = feedback #39(w661) -> (w690:dbl)
            n332 = feedback-in #39(w693) -> ()
            n333 = Divide(x=w675, y=25.4) -> (x/y=w673:dbl)
            n334 = feedback #40(w661) -> (w688:dbl)
            n335 = feedback-in #40(w690) -> ()
            n336 = Divide(x=w668, y=25.4) -> (x/y=w670:dbl)
            n337 = feedback #41(w661) -> (w687:dbl)
            n338 = feedback-in #41(w688) -> ()
            n339 = Multiply(x=w673, y=1000.0) -> (x*y=w666:dbl)
            n340 = feedback #42(w661) -> (w686:dbl)
            n341 = feedback-in #42(w687) -> ()
            n342 = Multiply(x=w670, y=1000.0) -> (x*y=w663:dbl)
            n343 = feedback-in #37(w663) -> ()
            n344 = feedback #43(w661) -> (w685:dbl)
            n345 = feedback-in #43(w686) -> ()
            n346 = feedback #44(w660) -> (w700:dbl)
            n347 = feedback-in #44(w666) -> ()
            n348 = feedback #45(w661) -> (w684:dbl)
            n349 = feedback-in #45(w685) -> ()
            n350 = feedback #46(w660) -> (w681:dbl)
            n351 = feedback #47(w661) -> (w683:dbl)
            n352 = Compound Arithmetic op=ADD(w663, w694, w693, w690, w688, w687, w686, w685, w684, w683) -> (w692:dbl)
            n353 = feedback-in #47(w684) -> ()
            n354 = feedback #48(w660) -> (w699:dbl)
            n355 = feedback-in #48(w700) -> ()
            n356 = feedback #49(w660) -> (w680:dbl)
            n357 = feedback-in #49(w681) -> ()
            n358 = feedback #50(w660) -> (w696:dbl)
            n359 = feedback-in #50(w699) -> ()
            n360 = feedback #51(w660) -> (w679:dbl)
            n361 = feedback-in #51(w680) -> ()
            n362 = feedback #52(w660) -> (w678:dbl)
            n363 = feedback-in #52(w679) -> ()
            n364 = feedback #53(w660) -> (w682:dbl)
            n365 = feedback-in #46(w682) -> ()
            n366 = feedback-in #53(w696) -> ()
            n367 = Divide(x=w692, y=10.0) -> (x/y=w689:dbl)
            n368 = feedback #54(w660) -> (w677:dbl)
            n369 = feedback-in #54(w678) -> ()
            n370 = call <vilib>:"Get_YPRHfH.vi"() -> ("YRPHfH"=w713:T17)  [unwired: 11 in]
            n371 = Bundle(w689) -> ()  [unwired: 1 in, 1 out]
            n372 = Unbundle By Name(w713) -> ("Yaw"=w705:dbl)
            n373 = Compound Arithmetic op=ADD(w666, w700, w699, w696, w682, w681, w680, w679, w678, w677) -> (w698:dbl)
            n374 = Divide(x=w698, y=10.0) -> (x/y=w695:dbl)
            n375 = Bundle(w695) -> ()  [unwired: 1 in, 1 out]
            n376 = call-poly <vilib>:"NT Read Value.vi"("Name"="dist limit") -> ("Numeric"=w658:dbl)  [unwired: 9 in, 1 out]
            "limit of sensor dist 3" <- w658
            n377 = Unbundle By Name("PID gains 3") -> ("proportional gain (Kc)"=→"proportional gain (Kc) 3":dbl, "integral time (Ti, min)"=→"integral time (Ti, min) 3":dbl, "derivative time (Td, min)"=→"derivative time (Td, min) 3":dbl)
            n378 = call-poly <vilib>:"PID.vi"("output range"=cluster{"output high":dbl, "output low":dbl} {"output high"=0.2, "output low"=-0.2}, "PID gains"="PID gains 3", "process variable"=w705, "setpoint"="setpoint 3") -> ("dt out (s)"=w714:dbl, "output"=w715:dbl)  [unwired: 6 in]
            n379 = Less?(x=w658, y=w695) -> (x < y?=w701:bool)
            "substitute 3" <- w701
            n380 = Less?(x=w658, y=w689) -> (x < y?=w721:bool)
            n381 = Subtract(x=w705, y="setpoint 3") -> (x-y=w709:dbl)
            n382 = Or(x=w701, y=w721) -> (x .or. y?=w720:bool)
            "x .or. y? 3" <- w720
            n383 = Absolute Value(x=w709) -> (abs(x)=w707:dbl)
            n384 = Bundle("setpoint 3"="setpoint 3", "Yaw"=w705, "dt out (s)"=w714) -> ()  [unwired: 1 in, 1 out]
            n385 = Not(x=w720) -> (.not. x?=w662:bool)
            "STOP? 3" <- w662
            n386 = Greater?(x=w707, y=3.0) -> (0:w710:bool)
            n387 = Select(t="speed 3", s=w720, f=0.0) -> (s? t:f=w722:dbl)
            "s? t:f 3" <- w722
            n388 = Select(t=w715, s=w710, f=0.0) -> (s? t:f=w706:dbl)
            n389 = call-poly <vilib>:"WPI_RobotDriveHolonomicDrive.vi"("Rotation"=w706, "Y"=w722, "X"=0.0, "RobotDriveDevRef"=w702) -> ("RobotDriveDevRef"=w703:T12)  [unwired: 5 in, 2 out]
          }
        }
        frame #4 {
          # "(For use with infrared sensors in the future)"
        }
        frame #5 {
          n390 = Wait (ms)(milliseconds to wait=u32 2000) -> ()  [unwired: 1 out]
        }
        frame #6 {
          n391 = call-poly <vilib>:"WPI_SolenoidSet.vi"("Value"=WPI_SolenoidValue."Forward", "SolenoidDevRef"=w735) -> ("SolenoidDevRef"=w734:T8)  [unwired: 8 in, 1 out]
        }
        frame #7 {
          n392 = while {
            tunnel: w739 -> [w745]
            tunnel: [w744] -> w738
            stop <- w741 stop-if-true
            # "y\nx"
            # "move back from lift"
            n393 = call <vilib>:"Get_YPRHfH.vi"() -> ("YRPHfH"=w755:T17)  [unwired: 11 in]
            n394 = Unbundle By Name(w755) -> ("Yaw"=w754:dbl)
            n395 = Subtract(x=w754, y=0.0) -> (x-y=w752:dbl)
            n396 = Absolute Value(x=w752) -> (abs(x)=w751:dbl)
            n397 = call-poly <vilib>:"PID.vi"("output range"=cluster{"output high":dbl, "output low":dbl} {"output high"=0.2, "output low"=-0.2}, "PID gains"=T1 {"proportional gain (Kc)"=0.284, "integral time (Ti, min)"=0.00243, "derivative time (Td, min)"=0.0}, "process variable"=w754, "setpoint"=0.0) -> ("output"=w747:dbl)  [unwired: 6 in, 1 out]
            n398 = call "Elapsed Time7"("Time Target (s)"=3.0) -> ("Elapsed Time (s)"=→"Elapsed Time (s) 3":dbl, "Time has Elapsed"=w741:bool)  [unwired: 11 in, 6 out]
            "Time has Elapsed 3" <- w741
            n399 = Greater?(x=w751, y=3.0) -> (0:w748:bool)
            n400 = Select(t=w747, s=w748, f=0.0) -> (s? t:f=w746:dbl)
            n401 = call-poly <vilib>:"WPI_RobotDriveHolonomicDrive.vi"("Rotation"=w746, "Y"=-0.1, "X"=0.0, "RobotDriveDevRef"=w745) -> ("RobotDriveDevRef"=w744:T12)  [unwired: 5 in, 2 out]
          }
          n402 = call-poly <vilib>:"WPI_SolenoidSet.vi"("Value"=WPI_SolenoidValue."Forward", "SolenoidDevRef"=w736) -> ()  [unwired: 8 in, 2 out]
        }
        frame #8 {
          # "right is -\nleft is +"
          # "we want it to go left"
          # "shifts left or right\n(tbh idk which)"
          n403 = while {
            tunnel: w761 -> [w766]
            tunnel: [w765] -> w760
            stop <- w762 stop-if-true
            # "y\nx"
            n404 = call <vilib>:"Get_YPRHfH.vi"() -> ("YRPHfH"=w776:T17)  [unwired: 11 in]
            n405 = Unbundle By Name(w776) -> ("Yaw"=w775:dbl)
            n406 = Subtract(x=w775, y=180.0) -> (x-y=w773:dbl)
            n407 = Absolute Value(x=w773) -> (abs(x)=w772:dbl)
            n408 = call-poly <vilib>:"PID.vi"("output range"=cluster{"output high":dbl, "output low":dbl} {"output high"=0.2, "output low"=-0.2}, "PID gains"=T1 {"proportional gain (Kc)"=0.284, "integral time (Ti, min)"=0.00243, "derivative time (Td, min)"=0.0}, "process variable"=w775, "setpoint"=0.0) -> ("output"=w768:dbl)  [unwired: 6 in, 1 out]
            n409 = Greater?(x=w772, y=3.0) -> (0:w769:bool)
            n410 = call "Elapsed Time8"("Time Target (s)"=5.0) -> ("Time has Elapsed"=w762:bool)  [unwired: 11 in, 7 out]
            n411 = Select(t=w768, s=w769, f=0.0) -> (s? t:f=w767:dbl)
            n412 = call-poly <vilib>:"WPI_RobotDriveHolonomicDrive.vi"("Rotation"=w767, "Y"=0.0, "X"=-0.5, "RobotDriveDevRef"=w766) -> ("RobotDriveDevRef"=w765:T12)  [unwired: 5 in, 2 out]
          }
        }
        frame #9 {
          n413 = call <vilib>:"Zero Yaw.vi"("Zero"=TRUE) -> ()  [unwired: 11 in]
        }
        frame #10 {
          # "forward again"
          n414 = while {
            tunnel: w783 -> [w788]
            tunnel: [w787] -> _
            stop <- w784 stop-if-true
            # "y\nx"
            n415 = call <vilib>:"Get_YPRHfH.vi"() -> ("YRPHfH"=w798:T17)  [unwired: 11 in]
            n416 = Unbundle By Name(w798) -> ("Yaw"=w797:dbl)
            n417 = Subtract(x=w797, y=0.0) -> (x-y=w795:dbl)
            n418 = Absolute Value(x=w795) -> (abs(x)=w794:dbl)
            n419 = call-poly <vilib>:"PID.vi"("output range"=cluster{"output high":dbl, "output low":dbl} {"output high"=0.2, "output low"=-0.2}, "PID gains"=T1 {"proportional gain (Kc)"=0.284, "integral time (Ti, min)"=0.00243, "derivative time (Td, min)"=0.0}, "process variable"=w797, "setpoint"=0.0) -> ("output"=w790:dbl)  [unwired: 6 in, 1 out]
            n420 = Greater?(x=w794, y=3.0) -> (0:w791:bool)
            n421 = call "Elapsed Time9"("Time Target (s)"=2.0) -> ("Time has Elapsed"=w784:bool)  [unwired: 11 in, 7 out]
            n422 = Select(t=w790, s=w791, f=0.0) -> (s? t:f=w789:dbl)
            n423 = call-poly <vilib>:"WPI_RobotDriveHolonomicDrive.vi"("Rotation"=w789, "Y"=0.1, "X"=0.0, "RobotDriveDevRef"=w788) -> ("RobotDriveDevRef"=w787:T12)  [unwired: 5 in, 2 out]
          }
        }
      }
    }
  }
